vi "Zaber A Series Raster Scan.vi"() -> ()   [LabVIEW 2013]
doc: "This VI is an application for doing raster scans or well plate traversals with Zaber stages. It can traverse a grid with any number of axes, and at each grid point can optionally send a sequence of commands to other Zaber devices, along with custom user-defined actions. \n\nYou must have at least two stages or a two-axis stage connected to your serial port to use this program."
uses:
  Zaber A Series.lvlib
panel:
  in  "Cluster":T1
  in  "Playback":enum32{"Page 2"}(tab)
  out "Progress":u8(slide) scale=0.0..100.0
  in  "Run":bool
  in  "Home All":bool
  in  "Stop":bool
  in  "Traversal Order":bool
  in  "Actions to Perform":enum32{"Page 2"}(tab)
  in  "Device and Axis for Action":string
  in  "Add Action":bool
  in  "Next Action":T2(radio)
  in  "Command":string
  in  "Delay in milliseconds":i32
  in  "Actions":T3(array[cluster])
  in  "Axis Order":enum32{"Page 2"}(tab)
  in  "Device and Axis":string
  in  "Start Position":dbl
  in  "End Position":dbl
  in  "Number of Stops":i32=1 min=1
  in  "Add Axis":bool
  in  "Units (0: microsteps)":u16(ring) items=["microsteps", "microns", "millimeters", "inches", "degrees"]
  in  "Microstep Size (0)":dbl
  in  "Axes":T4(array[cluster])
  in  "Close Port":bool
  out "Port open":bool
  in  "VISA resource name":refnum<visa-resource-name>
  in  "Open Port":bool
  in  "Quit":bool
  # "Serial Port"
  # "This example will orchestrate a raster scan on any number of axes, and optionally run a sequence of other commands at each increment of the scan."
  # "Open your the serial port at top left. Then in the middle panel, add two or more device axes to the list, specifying the number of stops for each axis at the same time. To reverse the direction of an axis, set the start position higher than the end position.\n \nThe first axis added will be the one that moves most often, and the last the least often.\n\nTo clear the list of axes and start over, right-click on the Axes list and select \"Empty array\"."
  # "You can optionally add a list of actions to be performed at each step. Select the action type and options; Device and axis are required for both the Send Command and Wait for Idle actions. Delay only needs the time to wait. A 'Custom' function is available, and a space is left in the block diagram for you to enter a desired action.\n\nDo not include the leading \"/\" in Zaber ASCII commands.\n\nTo clear the list of actions, right-click on the Actions list and select \"Empty array\".\n\nPress the \"Home All\" button before the first run, then \"Run\" to start."
  # "(c) 2017 Zaber Technologies.  ALL RIGHTS RESERVED."
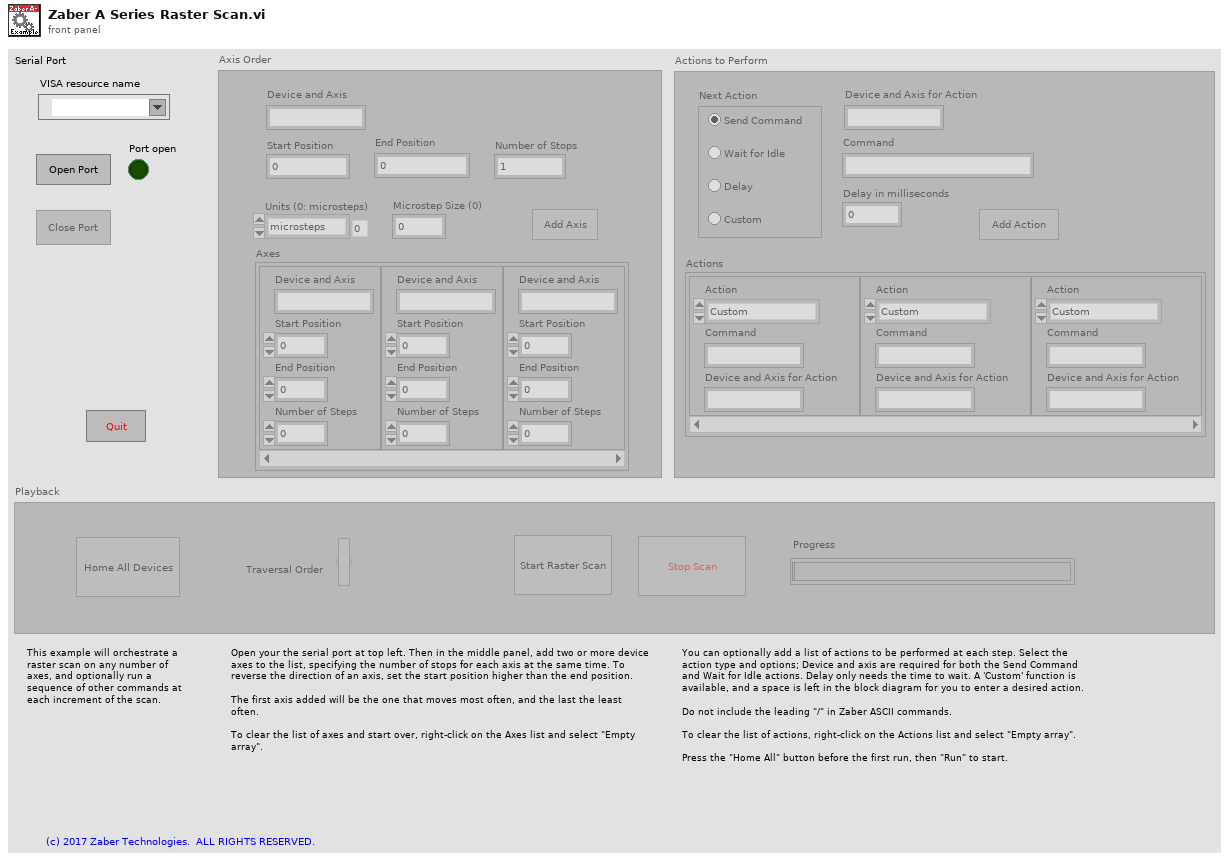
[diagram p1: front panel]
types:
  T1 = cluster{"Device and Axis":string, "Start Position":i64, "End Position":i64, "Number of Steps":i32}
  T2 = enum32{"Text Command Action", "Wait for Idle Action", "Delay Action", "Delay Action 2"}
  T3 = cluster{"Action":enum32{"Text Command Action", "Wait for Idle Action", "Delay Action", "Custom", ""}, "Command":string, "Device and Axis for Action":string}[]
  T4 = cluster{"Device and Axis":string, "Start Position":i64, "End Position":i64, "Number of Steps":i32}[]
  T5 = enum8{"Enabled", "Disabled", "Disabled and Grayed Out"}
  T6 = enum16{"Exiting", "Idling with port closed", "Opening port", "Closing port", "Idling with port open", "Add axis", "Add action", "Run sequence", "Home all axes"}
  T7 = cluster{"Next Action":enum32{"Text Command Action", "Wait for Idle Action", "Delay Action", "Delay Action 2"}, "Command":string, "Device and Axis for Action":string}
  T8 = cluster{"Next Action":u32, "Command":string, "Device and Axis for Action":string}[]
  T9 = enum32{"Text Command Action", "Wait for Idle Action", "Delay Action", "Custom", ""}
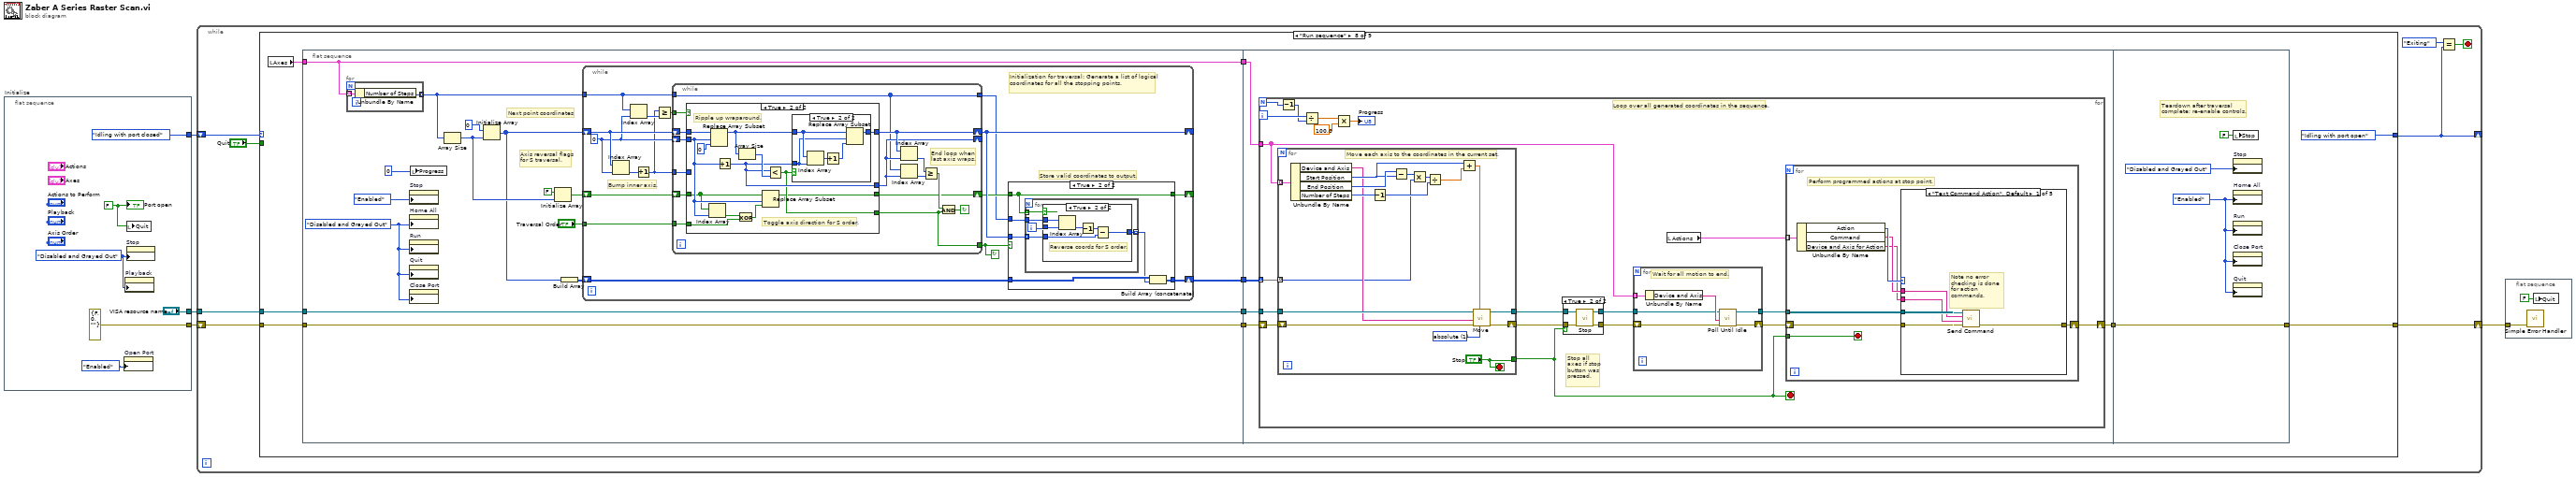
[diagram p0: block diagram]
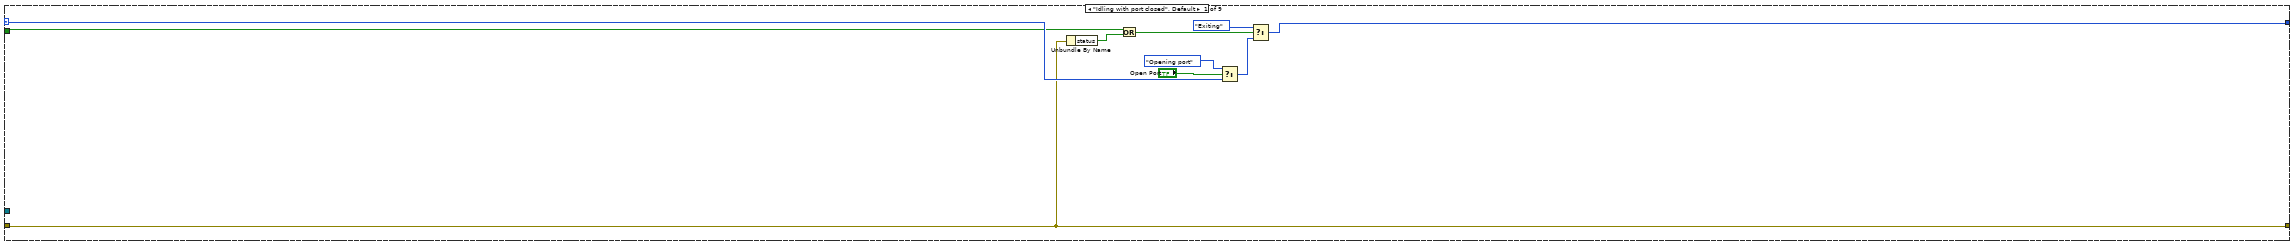
[diagram p2: hidden frame]
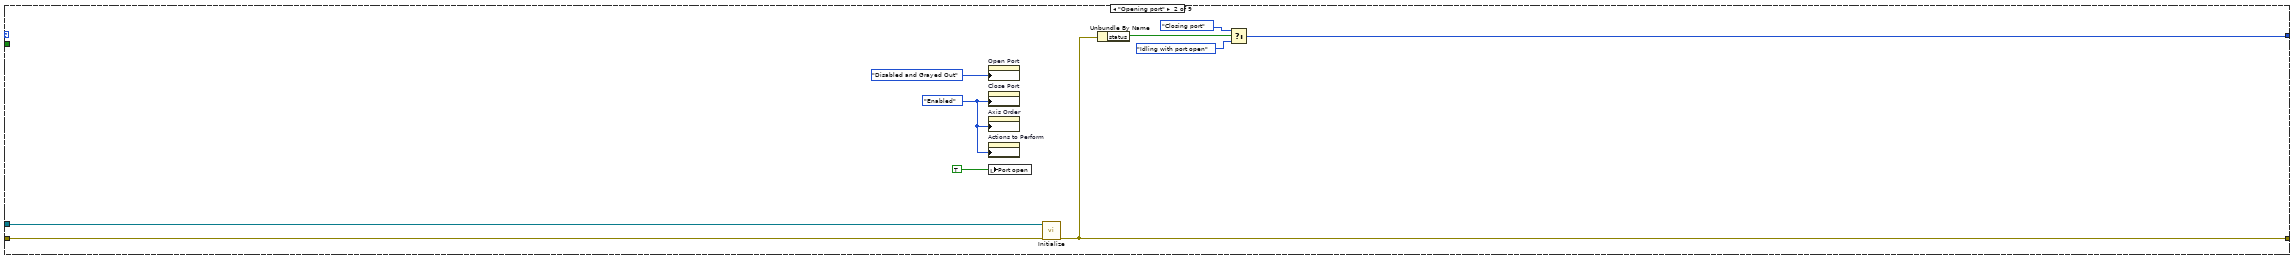
[diagram p3: hidden frame]
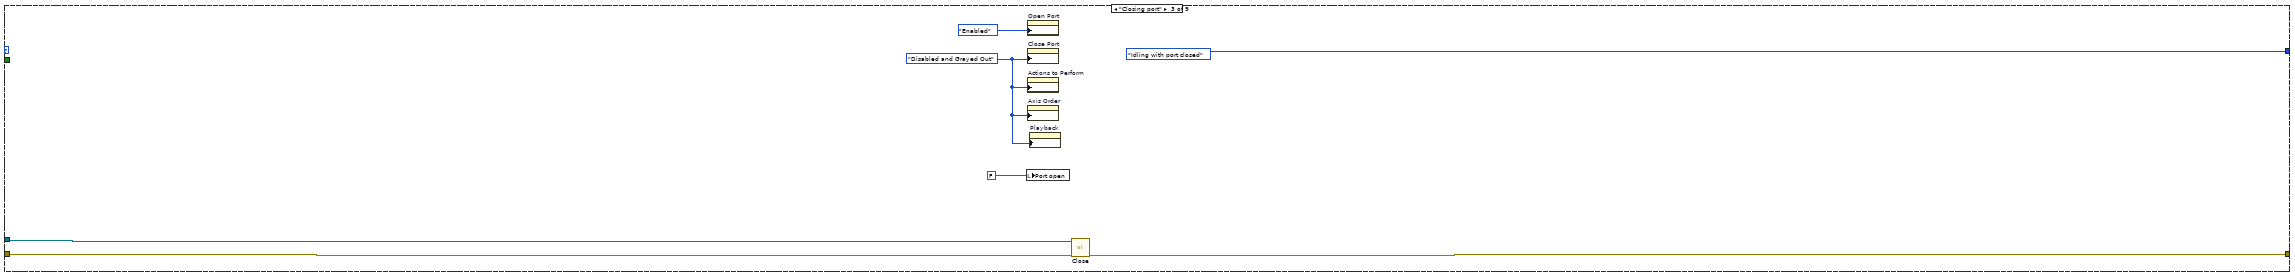
[diagram p4: hidden frame]
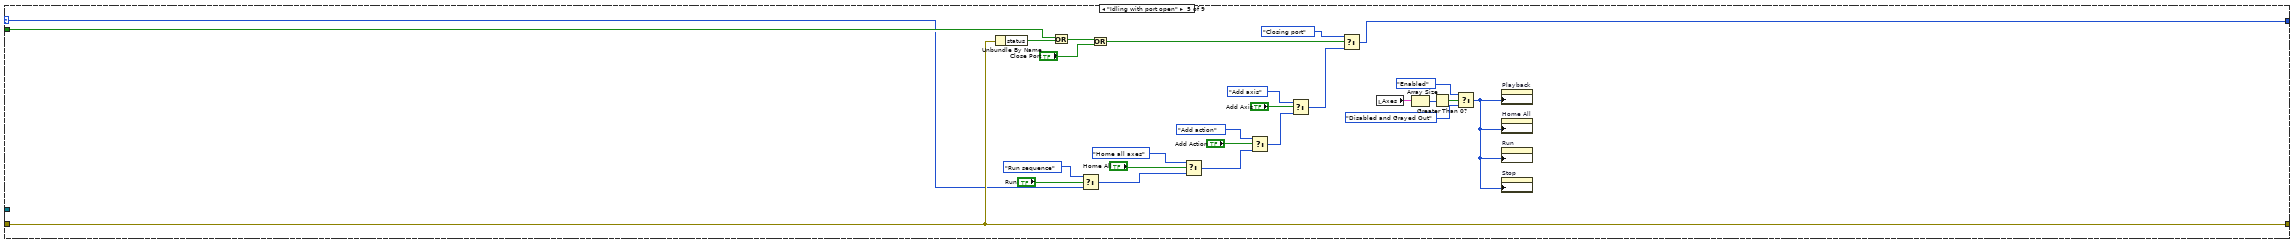
[diagram p6: hidden frame]
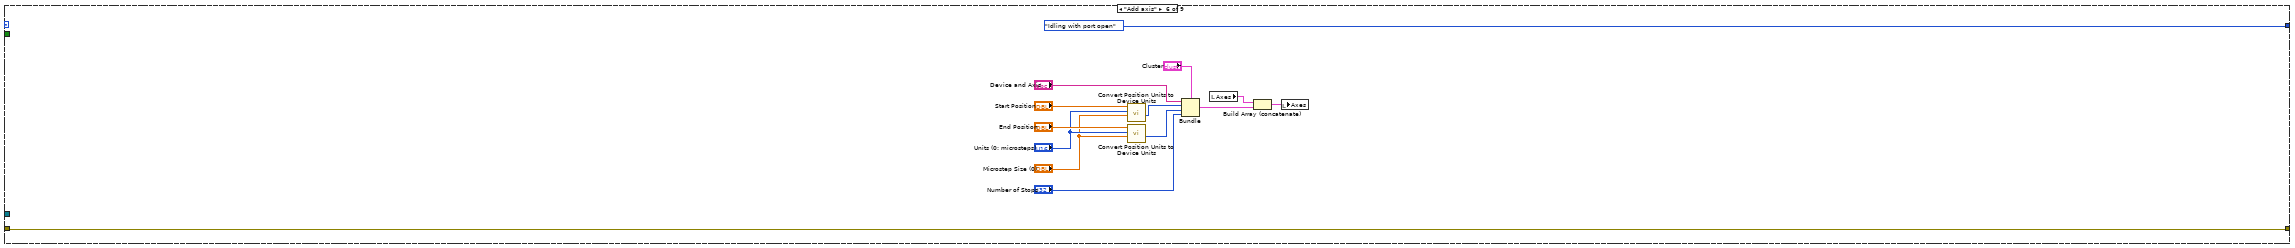
[diagram p7: hidden frame]
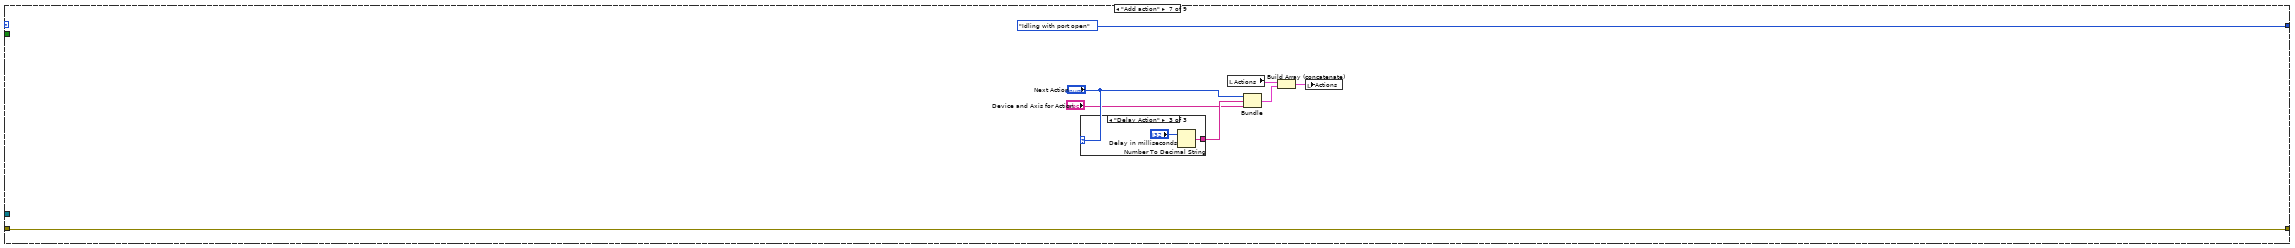
[diagram p8: hidden frame]
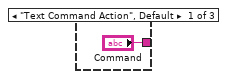
[diagram p9: hidden frame]
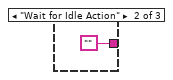
[diagram p10: hidden frame]
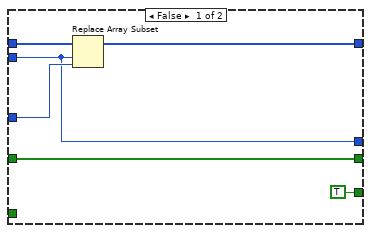
[diagram p13: hidden frame]
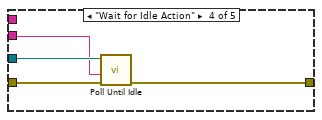
[diagram p17: hidden frame]
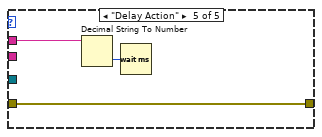
[diagram p18: hidden frame]
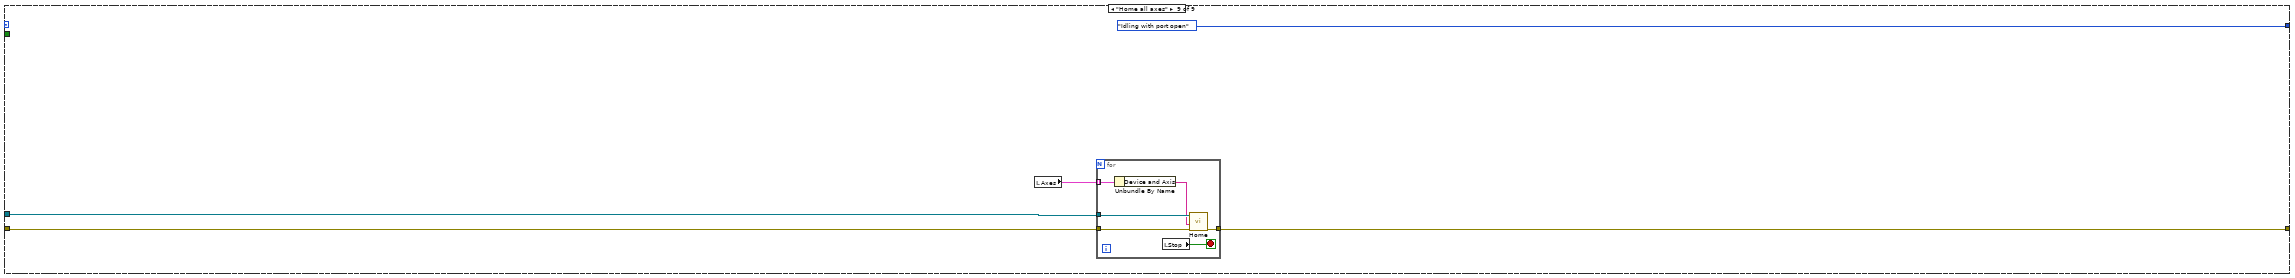
[diagram p20: hidden frame]
diagram:
  n1 = flat-sequence "Initialize" {
    tunnel: ["VISA resource name"] -> w4
    tunnel: [errorcluster {"status"=FALSE, "code"=0, "source"=""} ("error out")] -> w2
    tunnel: [T6."Idling with port closed"] -> w1
    frame #0 {
      w5 = T5."Disabled and Grayed Out" ("Disabled")
      w7 = FALSE ("Port open")
      n2 = property on="Open Port" class="Bool"("DisabledEnum"=T5."Enabled" ("Disabled")) -> ()  [unwired: 2 in, 2 out]
      n3 = property on="Playback" class="TabCtl (strict)"("DisabledEnum"=w5) -> ()  [unwired: 2 in, 2 out]
      n4 = local write "Quit"(w7) -> ()
      n5 = property on="Stop" class="Bool (strict)"("DisabledEnum"=w5) -> ()  [unwired: 2 in, 2 out]
      "Port open" <- w7
    }
  }
  n6 = while {
    tunnel: w4 -> [w16]
    shift-right: [w14] -> w3
    shift-left: w2 -> [w15]
    shift-right: [w12] -> _
    shift-left: w1 -> [w13]
    stop <- w18 stop-if-true
    n7 = case shown="\"Run sequence\"" w13 {
      selector: w13 -> [w28 _ _ w46 w52 _ _ _ _]
      tunnel: "Quit" -> [w24 _ _ _ w72 _ _ _ _]
      tunnel: w16 -> [_ w38 w44 _ _ _ _ w107 w286]
      tunnel: w15 -> [w25 w37 w45 w47 w74 w88 w96 w105 w285]
      tunnel: [w25 w36 w43 w47 w74 w88 w96 w104 w284] -> w14
      tunnel: [w21 w32 T6."Idling with port closed" w46 w68 T6."Idling with port open" T6."Idling with port open" T6."Idling with port open" ("t") T6."Idling with port open" ("t")] -> w12
      frame "Idling with port closed", Default {
        n8 = Unbundle By Name(w25) -> ("status"=w22:bool)
        n9 = Or(x=w24, y=w22) -> (x .or. y?=w23:bool)
        n10 = Select(t=T6."Opening port", s="Open Port", f=w28) -> (s? t:f=w27:T6)
        n11 = Select(t=T6."Exiting", s=w23, f=w27) -> (s? t:f=w21:T6)
      }
      frame "Opening port" {
        w31 = T5."Enabled" ("Disabled")
        n12 = property on="Open Port" class="Bool"("DisabledEnum"=T5."Disabled and Grayed Out" ("Disabled")) -> ()  [unwired: 2 in, 2 out]
        n13 = property on="Close Port" class="Bool"("DisabledEnum"=w31) -> ()  [unwired: 2 in, 2 out]
        n14 = property on="Axis Order" class="TabCtl (strict)"("DisabledEnum"=w31) -> ()  [unwired: 2 in, 2 out]
        n15 = property on="Actions to Perform" class="TabCtl (strict)"("DisabledEnum"=w31) -> ()  [unwired: 2 in, 2 out]
        n16 = local write "Port open"(TRUE ("Port open")) -> ()
        n17 = call "Initialize.vi"("error in (no error)"=w37, "VISA resource name"=w38) -> ("error out"=w36:errorcluster)  [unwired: 8 in, 1 out]
        n18 = Unbundle By Name(w36) -> ("status"=w35:bool)
        n19 = Select(t=T6."Closing port", s=w35, f=T6."Idling with port open") -> (s? t:f=w32:T6)
      }
      frame "Closing port" {
        w39 = T5."Disabled and Grayed Out" ("Disabled")
        n20 = local write "Port open"(FALSE ("Port open")) -> ()
        n21 = property on="Open Port" class="Bool"("DisabledEnum"=T5."Enabled" ("Disabled")) -> ()  [unwired: 2 in, 2 out]
        n22 = property on="Close Port" class="Bool"("DisabledEnum"=w39) -> ()  [unwired: 2 in, 2 out]
        n23 = property on="Actions to Perform" class="TabCtl (strict)"("DisabledEnum"=w39) -> ()  [unwired: 2 in, 2 out]
        n24 = property on="Axis Order" class="TabCtl (strict)"("DisabledEnum"=w39) -> ()  [unwired: 2 in, 2 out]
        n25 = property on="Playback" class="TabCtl (strict)"("DisabledEnum"=w39) -> ()  [unwired: 2 in, 2 out]
        n26 = call "Close.vi"("error in (no error)"=w45, "VISA resource name"=w44) -> ("error out"=w43:errorcluster)  [unwired: 9 in]
      }
      frame "Exiting" {
      }
      frame "Idling with port open" {
        n27 = Unbundle By Name(w74) -> ("status"=w73:bool)
        n28 = Or(x=w72, y=w73) -> (x .or. y?=w71:bool)
        n29 = Select(t=T6."Run sequence", s="Run", f=w52) -> (s? t:f=w51:T6)
        n30 = Or(x=w71, y="Close Port") -> (x .or. y?=w69:bool)
        n31 = Select(t=T6."Home all axes", s="Home All", f=w51) -> (s? t:f=w55:T6)
        n32 = Select(t=T6."Add action", s="Add Action", f=w55) -> (s? t:f=w67:T6)
        n33 = Select(t=T6."Add axis", s="Add Axis", f=w67) -> (s? t:f=w66:T6)
        n34 = Select(t=T6."Closing port", s=w69, f=w66) -> (s? t:f=w68:T6)
        n35 = local read "Axes"() -> (w60:T4)
        n36 = Array Size(array=w60) -> (size(s)=w59:i32)
        n37 = Greater Than 0?(x=w59) -> (x > 0?=w58:bool)
        n38 = Select(t=T5."Enabled" ("Disabled"), s=w58, f=T5."Disabled and Grayed Out") -> (s? t:f=w48:T5)
        n39 = property on="Playback" class="TabCtl (strict)"("DisabledEnum"=w48) -> ()  [unwired: 2 in, 2 out]
        n40 = property on="Home All" class="Bool"("DisabledEnum"=w48) -> ()  [unwired: 2 in, 2 out]
        n41 = property on="Run" class="Bool"("DisabledEnum"=w48) -> ()  [unwired: 2 in, 2 out]
        n42 = property on="Stop" class="Bool (strict)"("DisabledEnum"=w48) -> ()  [unwired: 2 in, 2 out]
      }
      frame "Add axis" {
        n43 = call "Convert Position Units to Device Units.vi"("Microstep Size (0)"="Microstep Size (0)", "Units (0: microsteps)"="Units (0: microsteps)", "Position (0)"="Start Position") -> ("Device Position (64-bit)"=w76:i64)  [unwired: 6 in, 2 out]
        n44 = call "Convert Position Units to Device Units.vi"("Microstep Size (0)"="Microstep Size (0)", "Units (0: microsteps)"="Units (0: microsteps)", "Position (0)"="End Position") -> ("Device Position (64-bit)"=w75:i64)  [unwired: 6 in, 2 out]
        n45 = Bundle(cluster="Cluster", "Device and Axis"="Device and Axis", "Start Position"=w76, "End Position"=w75, "Number of Steps"="Number of Stops") -> (w82:T1)
        n46 = local read "Axes"() -> (w87:T4)
        n47 = Build Array (concatenate)(w87, w82) -> (w77:T4)
        n48 = local write "Axes"(w77) -> ()
      }
      frame "Add action" {
        n49 = case shown="\"Delay Action\"" "Next Action" {
          tunnel: ["Command" "" w99] -> w93
          frame "Text Command Action", Default {
          }
          frame "Wait for Idle Action" {
          }
          frame "Delay Action" {
            n50 = Number To Decimal String(number="Delay in milliseconds") -> (decimal integer string=w99:string)  [unwired: 1 in]
          }
        }
        n51 = local read "Actions"() -> (w90:T3)
        n52 = Bundle("Next Action"="Next Action", "Command"=w93, "Device and Axis for Action"="Device and Axis for Action") -> (w91:T7)  [unwired: 1 in]
        n53 = Build Array (concatenate)(w90, w91) -> (w89:T8)
        n54 = local write "Actions"(w89) -> ()
      }
      frame "Run sequence" {
        n55 = local read "Axes"() -> (w110:T4)
        n56 = flat-sequence {
          tunnel: w110 -> [w121]
          tunnel: [w121] -> w109
          tunnel: [w124] -> w108
          tunnel: w107 -> [w124]
          tunnel: [w123] -> w106
          tunnel: w105 -> [w123]
          tunnel: [w113] -> w101
          tunnel: w109 -> [w208]
          tunnel: w108 -> [w207]
          tunnel: w106 -> [w206]
          tunnel: [w204] -> w103
          tunnel: w101 -> [w205]
          tunnel: [w281] -> w104
          tunnel: w103 -> [w281]
          frame #0 {
            w122 = T5."Disabled and Grayed Out" ("Disabled")
            # "Axis reversal flags\nfor S traversal."
            # "Next point coordinates"
            n57 = for {
              tunnel: w121 -> [w127] mode=indexing
              tunnel: [w126] -> w117 mode=indexing
              n58 = Unbundle By Name(w127) -> ("Number of Steps"=w126:i32)
            }
            n59 = property on="Stop" class="Bool (strict)"("DisabledEnum"=T5."Enabled" ("Disabled")) -> ()  [unwired: 2 in, 2 out]
            n60 = property on="Home All" class="Bool"("DisabledEnum"=w122) -> ()  [unwired: 2 in, 2 out]
            n61 = property on="Run" class="Bool"("DisabledEnum"=w122) -> ()  [unwired: 2 in, 2 out]
            n62 = property on="Quit" class="Bool (strict)"("DisabledEnum"=w122) -> ()  [unwired: 2 in, 2 out]
            n63 = property on="Close Port" class="Bool"("DisabledEnum"=w122) -> ()  [unwired: 2 in, 2 out]
            n64 = local write "Progress"(u8 0 ("Progress")) -> ()
            n65 = Array Size(array=w117) -> (size(s)=w119:i32)
            n66 = Initialize Array(0, w119) -> (w116:i32[])
            n67 = Initialize Array(FALSE, w119) -> (w115:bool[])
            n68 = Build Array(w116) -> (w114:i32[][])
            n69 = while {
              tunnel: w117 -> [w134]
              shift-right: [w136] -> w113
              shift-left: w114 -> [w137]
              shift-right: [w135] -> _
              shift-left: w116 -> [w140]
              shift-right: [w129] -> _
              shift-left: w115 -> [w132]
              tunnel: "Traversal Order" -> [w131]
              stop <- w133 continue-if-true
              w139 = 0
              # "Initialization for traversal: Generate a list of logical coordinates for all the stopping points."
              # "Store valid coordinates to output."
              # "Bump inner axis."
              n70 = Index Array(array=w140, index=w139) -> (element=w143:i32)
              n71 = Index Array(array=w134, index=w139) -> (element=w142:i32)
              n72 = Increment(x=w143) -> (x+1=w138:i32)
              n73 = Greater Or Equal?(x=w138, y=w142) -> (x >= y?=w141:bool)
              n74 = while {
                tunnel: w141 -> [w178]
                tunnel: w138 -> [w175]
                shift-right: [w172] -> w135
                shift-left: w140 -> [w177]
                tunnel: [w173] -> w133
                shift-right: [w169] -> _
                shift-left: w139 -> [w176]
                tunnel: w134 -> [w164]
                shift-right: [w165] -> w130
                shift-left: w132 -> [w167]
                tunnel: w131 -> [w166]
                tunnel: [w164] -> w128
                stop <- w174 continue-if-true
                # "End loop when\nlast axis wraps."
                n75 = case shown="True" w178 {
                  tunnel: w177 -> [w184 w197]
                  tunnel: w176 -> [w181 w190]
                  tunnel: w175 -> [w183 _]
                  tunnel: [w182 w191] -> w172
                  tunnel: [TRUE w192] -> w173
                  tunnel: [w181 w193] -> w169
                  tunnel: w167 -> [w179 w189]
                  tunnel: w166 -> [_ w186]
                  tunnel: [w179 w185] -> w165
                  frame False {
                    n76 = Replace Array Subset(array=w184, new element=w183, index=w181) -> (w182:i32[])
                  }
                  frame True {
                    # "Toggle axis direction for S order."
                    # "Ripple up wraparound."
                    n77 = Index Array(array=w189, index=w190) -> (element=w187:bool)
                    n78 = Replace Array Subset(array=w197, new element=0 ("new element/subarray"), index=w190) -> (w194:i32[])
                    n79 = Increment(x=w190) -> (x+1=w193:i32)
                    n80 = Exclusive Or(1:w186, 2:w187) -> (0:w188:bool)
                    n81 = Array Size(array=w194) -> (size(s)=w195:i32)
                    n82 = Replace Array Subset(array=w189, new element=w188, index=w190) -> (w185:bool[])
                    n83 = Less?(x=w193, y=w195) -> (x < y?=w192:bool)
                    n84 = case shown="True" w192 {
                      tunnel: w194 -> [w198 w202]
                      tunnel: [w198 w203] -> w191
                      tunnel: w193 -> [_ w201]
                      frame False {
                      }
                      frame True {
                        n85 = Index Array(array=w202, index=w201) -> (element=w199:i32)
                        n86 = Increment(x=w199) -> (x+1=w200:i32)
                        n87 = Replace Array Subset(array=w202, new element=w200, index=w201) -> (w203:i32[])
                      }
                    }
                  }
                }
                n88 = Index Array(array=w172, index=w169) -> (element=w171:i32)
                n89 = Index Array(array=w164, index=w169) -> (element=w168:i32)
                n90 = Greater Or Equal?(x=w171, y=w168) -> (x >= y?=w170:bool)
                n91 = And(x=w170, y=w173) -> (x .and. y?=w174:bool)
              }
              n92 = case shown="True" w133 {
                tunnel: w137 -> [w145 w151]
                tunnel: [w145 w150] -> w136
                tunnel: w135 -> [_ w149]
                tunnel: w130 -> [w144 w147]
                tunnel: [w144 w147] -> w129
                tunnel: w128 -> [_ w146]
                frame False {
                }
                frame True {
                  n93 = for {
                    tunnel: w149 -> [w156] mode=indexing
                    tunnel: [w155] -> w148 mode=indexing
                    tunnel: w147 -> [w154] mode=indexing
                    tunnel: w146 -> [w153]
                    i -> [w152]
                    n94 = case shown="True" w154 {
                      tunnel: w156 -> [w157 w158]
                      tunnel: [w157 w159] -> w155
                      tunnel: w153 -> [_ w163]
                      tunnel: w152 -> [_ w162]
                      frame False {
                      }
                      frame True {
                        # "Reverse coords for S order."
                        n95 = Index Array(array=w163, index=w162) -> (element=w161:i32)
                        n96 = Decrement(x=w161) -> (x-1=w160:i32)
                        n97 = Subtract(x=w160, y=w158) -> (x-y=w159:i32)
                      }
                    }
                  }
                  n98 = Build Array (concatenate)(w151, w148) -> (w150:i32[][])
                }
              }
            }
          }
          frame #1 {
            n99 = for {
              N -> [w212]
              tunnel: w208 -> [w217]
              tunnel: w207 -> [w221]
              tunnel: w205 -> [w222] mode=indexing
              shift-right: [w209] -> w204
              shift-left: w206 -> [w220]
              i -> [w216]
              stop <- w210 stop-if-true
              # "Loop over all generated coordinates in the sequence."
              # "Stop all\naxes if stop\nbutton was\npressed."
              n100 = for {
                tunnel: w217 -> [w244] mode=indexing
                tunnel: w222 -> [w228] mode=indexing
                tunnel: w221 -> [w238]
                tunnel: [w232] -> w218
                tunnel: ["Stop"] -> w210
                shift-right: [w233] -> w219
                shift-left: w220 -> [w236]
                stop <- "Stop" stop-if-true
                w234 = u16 1 items=["relative", "absolute"] ("Movement Type (0: relative)")
                # "Move each axis to the coordinates in the current set."
                n101 = Unbundle By Name(w244) -> ("Device and Axis"=w235:string, "Start Position"=w241:i64, "End Position"=w243:i64, "Number of Steps"=w239:i32)
                n102 = Decrement(x=w239) -> (x-1=w230:i32)
                n103 = Subtract(x=w243, y=w241) -> (x-y=w242:i64)
                n104 = Multiply(x=w242, y=w228) -> (x*y=w240:i64)
                n105 = Divide(x=w240, y=w230) -> (x/y=w229:dbl)
                n106 = Add(x=w241, y=w229) -> (x+y=w237:dbl)
                n107 = call "Move.vi"("Movement Type (0: relative)"=w234, "Move Distance (0)"=w237, "error in (no error)"=w236, "Device and Axis"=w235, "VISA resource name"=w238) -> ("error out"=w233:errorcluster, "VISA resource name out"=w232:refnum<visa-resource-name>)  [unwired: 5 in]
              }
              n108 = Decrement(x=w212) -> (x-1=w211:i32)
              n109 = Divide(x=w216, y=w211) -> (x/y=w215:dbl)
              n110 = Multiply(x=w215, y=100.0) -> (x*y=→"Progress":dbl)
              n111 = case shown="True" w210 {
                tunnel: w218 -> [w268 w272]
                tunnel: [w268 w270] -> w227
                tunnel: w219 -> [w267 w271]
                tunnel: [w267 w269] -> w226
                frame False {
                }
                frame True {
                  n112 = call "Stop.vi"("error in (no error)"=w271, "VISA resource name"=w272) -> ("error out"=w269:errorcluster, "VISA resource name out"=w270:refnum<visa-resource-name>)  [unwired: 8 in]
                }
              }
              n113 = for {
                tunnel: w217 -> [w278] mode=indexing
                tunnel: w227 -> [w276]
                tunnel: [w274] -> w224
                shift-right: [w273] -> w223
                shift-left: w226 -> [w275]
                # "Wait for all motion to end."
                n114 = Unbundle By Name(w278) -> ("Device and Axis"=w277:string)
                n115 = call "Poll Until Idle.vi"("error in (no error)"=w275, "Device and Axis"=w277, "VISA resource name"=w276) -> ("error out"=w273:errorcluster, "VISA resource name out"=w274:refnum<visa-resource-name>)  [unwired: 7 in]
              }
              n116 = local read "Actions"() -> (w225:T3)
              n117 = for {
                tunnel: w225 -> [w252] mode=indexing
                tunnel: w224 -> [w249]
                tunnel: w210 -> [w246]
                shift-right: [w247] -> w209
                shift-left: w223 -> [w248]
                stop <- w246 stop-if-true
                # "Perform programmed actions at stop point."
                n118 = Unbundle By Name(w252) -> ("Action"=w251:T9, "Command"=w250:string, "Device and Axis for Action"=w245:string)
                n119 = case shown="\"Text Command Action\", Default" w251 {
                  tunnel: w250 -> [w254 _ _ _ w265]
                  tunnel: w249 -> [w257 _ _ w263 _]
                  tunnel: w248 -> [w256 w258 w259 w262 w266]
                  tunnel: [w255 w258 w259 w261 w266] -> w247
                  tunnel: w245 -> [w253 _ _ w260 _]
                  frame "Text Command Action", Default {
                    # "Note no error checking is done\nfor action commands."
                    n120 = call "Send Command.vi"("error in (no error)"=w256, "Device and Axis"=w253, "Command"=w254, "VISA resource name"=w257) -> ("error out"=w255:errorcluster)  [unwired: 2 in, 5 out]
                  }
                  frame "Custom" {
                    # "Enter your own custom actions to perform here."
                  }
                  frame "" {
                    # "This space intentionally left blank."
                  }
                  frame "Wait for Idle Action" {
                    n121 = call "Poll Until Idle.vi"("error in (no error)"=w262, "Device and Axis"=w260, "VISA resource name"=w263) -> ("error out"=w261:errorcluster)  [unwired: 7 in, 1 out]
                  }
                  frame "Delay Action" {
                    n122 = Decimal String To Number(string=w265) -> (number=w264:i32)  [unwired: 2 in, 1 out]
                    n123 = Wait (ms)(milliseconds to wait=w264) -> ()  [unwired: 1 out]
                  }
                }
              }
            }
          }
          frame #2 {
            w279 = T5."Enabled" ("Disabled")
            # "Teardown after traversal\ncomplete; re-enable controls."
            n124 = local write "Stop"(FALSE ("Stop")) -> ()
            n125 = property on="Stop" class="Bool (strict)"("DisabledEnum"=T5."Disabled and Grayed Out" ("Disabled")) -> ()  [unwired: 2 in, 2 out]
            n126 = property on="Home All" class="Bool"("DisabledEnum"=w279) -> ()  [unwired: 2 in, 2 out]
            n127 = property on="Run" class="Bool"("DisabledEnum"=w279) -> ()  [unwired: 2 in, 2 out]
            n128 = property on="Close Port" class="Bool"("DisabledEnum"=w279) -> ()  [unwired: 2 in, 2 out]
            n129 = property on="Quit" class="Bool (strict)"("DisabledEnum"=w279) -> ()  [unwired: 2 in, 2 out]
          }
        }
      }
      frame "Home all axes" {
        n130 = local read "Axes"() -> (w287:T4)
        n131 = for {
          tunnel: w287 -> [w293] mode=indexing
          tunnel: w286 -> [w291]
          tunnel: w285 -> [w290]
          tunnel: [w289] -> w284
          stop <- w292 stop-if-true
          n132 = Unbundle By Name(w293) -> ("Device and Axis"=w288:string)
          n133 = local read "Stop"() -> (w292:bool)
          n134 = call "Home.vi"("error in (no error)"=w290, "Device and Axis"=w288, "VISA resource name"=w291) -> ("error out"=w289:errorcluster)  [unwired: 7 in, 1 out]
        }
      }
    }
    n135 = Equal?(x=T6."Exiting", y=w12) -> (x = y?=w18:bool)
  }
  n136 = flat-sequence {
    tunnel: w3 -> [w295]
    frame #0 {
      n137 = call <vilib>:"Simple Error Handler.vi"("error in (no error)"=w295) -> ()  [unwired: 4 in, 5 out]
      n138 = local write "Quit"(FALSE ("Quit")) -> ()
    }
  }
